vi "GFITS_GetGeometryHeaders.vi"(9 "readmode":string) -> (3 "Keywords out":string[][][](array[string]))   [LabVIEW 2016]
panel:
  in  "geometry":string[][](table)
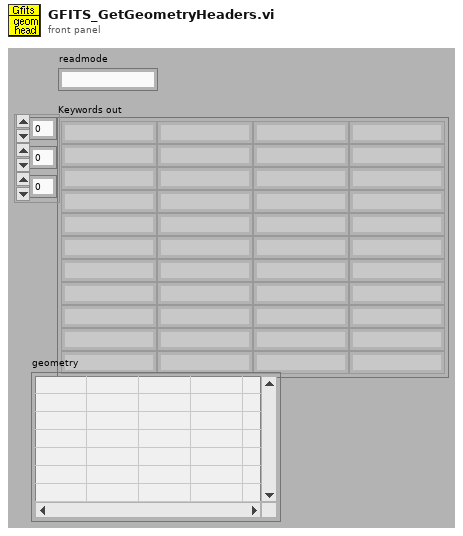
[diagram p1: front panel]
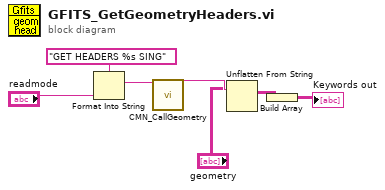
[diagram p0: block diagram]
diagram:
  n1 = Format Into String(format string="GET HEADERS %s SING" ("Command"), "readmode") -> (resulting string=w7:string)  [unwired: 2 in, 1 out]
  n2 = call "CMN_CallGeometry.vi"("Command"=w7) -> ("ImmedReplyString"=w6:string)  [unwired: 1 in, 13 out]
  n3 = Unflatten From String(type="geometry", binary string=w6) -> (value=w2:string[][])  [unwired: 1 in, 4 out]
  n4 = Build Array(w2) -> (→"Keywords out":string[][][])
